vi "ex4d.vi"() -> ()   [LabVIEW 2022 SP3]
panel:
  out "Seconds Counted":string
  in  "?":bool
  out "Seconds Counted":dbl caption="Elapsed Time (s)"
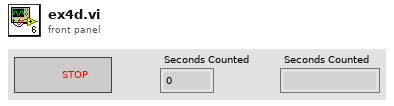
[diagram p1: front panel]
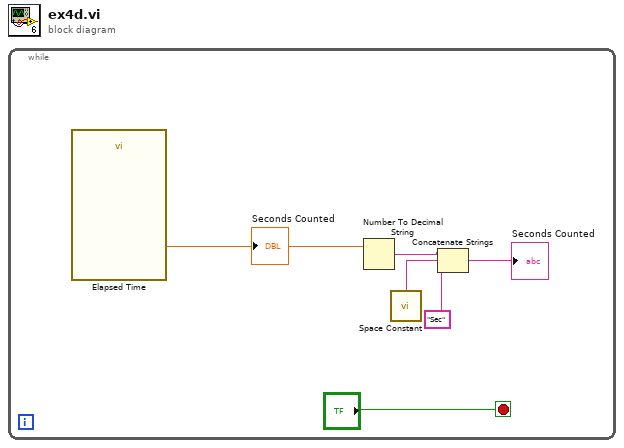
[diagram p0: block diagram]
diagram:
  n1 = while {
    stop <- "?" stop-if-true
    n2 = call "Elapsed Time"() -> ("Elapsed Time (s)"=w5:dbl)  [unwired: 12 in, 7 out]
    "Seconds Counted" <- w5
    n3 = Number To Decimal String(number=w5) -> (decimal integer string=w4:string)  [unwired: 1 in]
    n4 = call <vilib>:"Space Constant.vi"() -> ("String"=w3:string)
    n5 = Concatenate Strings(w4, w3, "Sec" ("string")) -> (→"Seconds Counted":string)
  }
